vi "CreateSMGR_01_file_old.vi"(7 "file path to write":path, 8 "error in":errorcluster, 10 "Waveform Graph":waveform(i16)[](graph), 11 "meas_point":i32=4) -> (0 "error out":errorcluster, 1 "microseconds str":string, 2 "date str":string, 3 "file path out":path, 4 "max_values":string[](array[string]))   [LabVIEW 2010]
panel:
  out "dt":dbl format="%#_6f"
  out "max_value str":string
  # "Записываем данные в смешанном виде (текстовый/бинарный)\n-------------------------------------------------------------------------------\nСправка по формату лежит здесь\nhttp://smgr-devel.alwaysdata.net/doku.php?id=start\n\nЕсли включен дебаг, то в файл записываются две синусоиды\nа время ставится текущее"
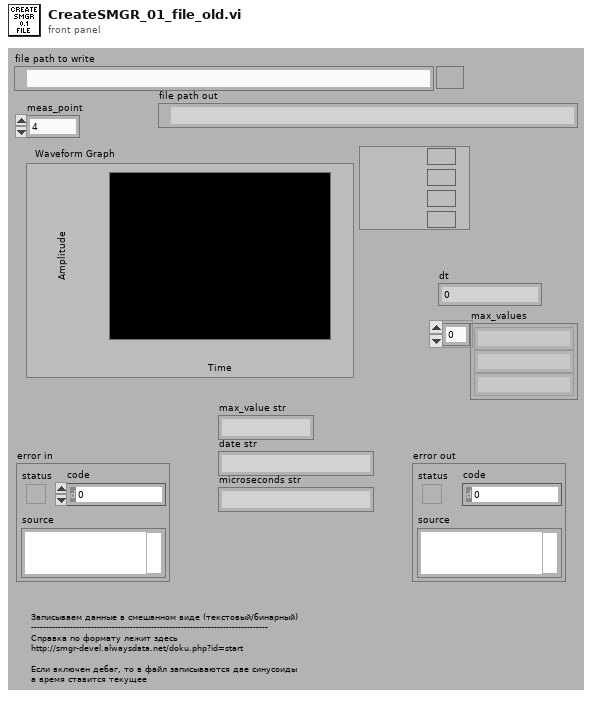
[diagram p1: front panel]
types:
  T1 = enum16{"sync", "phase_a", "phase_b", "phase_c", "ground"}
  T2 = enum16{"big-endian, network order", "native, host order", "little-endian"}
  T3 = enum16{"open", "replace", "create", "open or create", "replace or create", "replace or create with confirmation"}
  T4 = typedef "LVDateTimeRec.ctl" = cluster{"fractional second":dbl, "second":i32, "minute":i32, "hour":i32, "day of month":i32, "month":i32, "year":i32, "day of week":i32, "day of year":i32, "DST":i32}
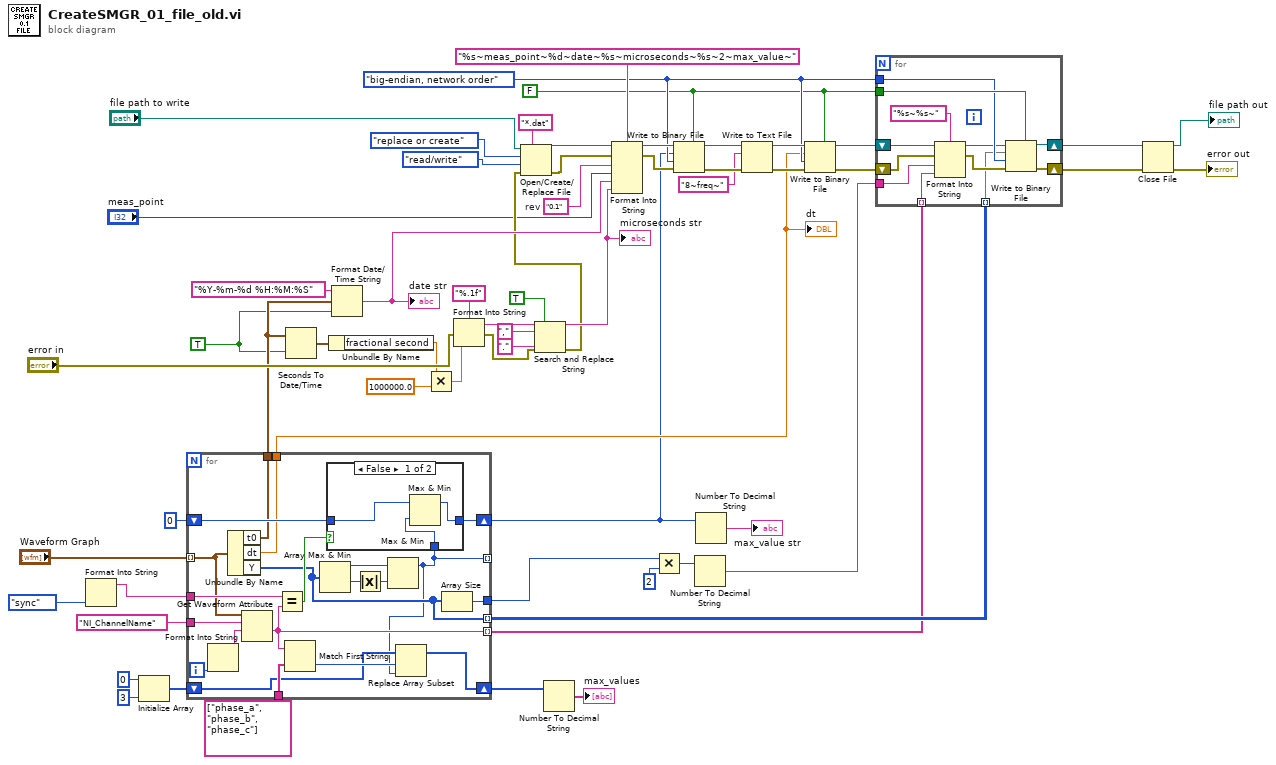
[diagram p0: block diagram]
diagram:
  w9 = TRUE ("to UTC (F)")
  w50 = "0.1"  # rev
  w39 = FALSE ("prepend array or string size? (T)")
  w40 = T2."big-endian, network order" ("byte order (0:big-endian, network order)")
  n1 = Format Into String(T1."sync") -> (resulting string=w16:string)  [unwired: 3 in, 1 out]
  n2 = Initialize Array(i16 0 ("element"), 3 ("dimension size")) -> (w4:i16[])
  n3 = for {
    tunnel: "Waveform Graph" -> [w78] mode=indexing
    tunnel: [w68] -> w41 mode=indexing
    tunnel: [w66] -> w8 mode=indexing
    shift-right: [w79] -> w3
    shift-left: i16 0 -> [w82]
    tunnel: w16 -> [w81]
    tunnel: "NI_ChannelName" -> [w77]
    tunnel: [w74] -> w15
    tunnel: [w73] -> w14
    tunnel: [w72] -> w13
    tunnel: [w62] -> _ mode=indexing
    tunnel: string[] ["phase_a", "phase_b", "phase_c"] -> [w67]
    shift-right: [w63] -> w2
    shift-left: w4 -> [w64]
    i -> [w76]
    n4 = Format Into String(w76) -> (resulting string=w75:string)  [unwired: 3 in, 1 out]
    n5 = Unbundle By Name(w78) -> ("t0"=w73:timestamp, "dt"=w74:dbl, "Y"=w68:i16[])
    n6 = Get Waveform Attribute(5:w75, 6:w77, 7:w78) -> (1:w66:string)  [unwired: 1 in, 3 out]
    n7 = Equal?(x=w81, y=w66) -> (x = y?=w80:bool)
    n8 = Match First String(2:w67, 3:w66) -> (0:w65:i32)  [unwired: 1 out]
    n9 = Array Max & Min(array=w68) -> (max value=w70:i16, min value=w69:i16)  [unwired: 2 out]
    n10 = Absolute Value(x=w69) -> (abs(x)=w71:i16)
    n11 = Max & Min(x=w70, y=w71) -> (max(x,y)=w62:i16)  [unwired: 1 out]
    n12 = case shown="False" w80 {
      tunnel: w82 -> [w84 w86]
      tunnel: [w85 w86] -> w79
      tunnel: w62 -> [w83 _]
      frame False {
        n13 = Max & Min(x=w84, y=w83) -> (max(x,y)=w85:i16)  [unwired: 1 out]
      }
      frame True {
      }
    }
    n14 = Replace Array Subset(array=w64, new element=w62, index=w65) -> (w63:i16[])
    n15 = Array Size(array=w68) -> (size(s)=w72:i32)
  }
  "dt" <- w15
  n16 = Seconds To Date/Time(time stamp (now)=w14, to UTC (F)=w9) -> (date time rec=w52:T4)
  n17 = Unbundle By Name(w52) -> ("fractional second"=w24:dbl)
  n18 = Format Date/Time String(time format string (%c)="%Y-%m-%d %H:%M:%S", seconds (now)=w14, UTC format=w9) -> (date/time string=w49:string)
  "date str" <- w49
  n19 = Multiply(x=w24, y=1000000.0) -> (x*y=w22:dbl)
  n20 = Format Into String(format string="%.1f", error in="error in", w22) -> (resulting string=w33:string, error out=w31:errorcluster)  [unwired: 1 in]
  n21 = Search and Replace String(replace all?=TRUE ("replace all? (F)"), input string=w33, search string=",", replace string="." ("replace string (\"\")"), error in=w31) -> (result string=w27:string, error out=w26:errorcluster)  [unwired: 3 in, 2 out]
  "microseconds str" <- w27
  n22 = Open/Create/Replace File(file path (use dialog)="file path to write", error in=w26, prompt="*.dat", operation (0:open)=T3."replace or create", access (0:read/write)=enum16{"read/write", "read-only", "write-only"}."read/write") -> (refnum out=w57:refnum<file>, error out=w56:errorcluster)  [unwired: 1 in, 1 out]
  n23 = Number To Decimal String(number=w2) -> (decimal integer string=→"max_values":string[])  [unwired: 1 in]
  n24 = Format Into String(format string="%s~meas_point~%d~date~%s~microseconds~%s~2~max_value~", initial string=w57, error in=w56, w50, "meas_point", w49, w27) -> (resulting string=w55:refnum<file>, error out=w54:errorcluster)
  n25 = Multiply(x=w13, y=2 ("index")) -> (x*y=w37:i32)
  n26 = Write to Binary File(file (use dialog)=w55, data=w3, error in=w54, 5:w39, 9:w40) -> (refnum out=w47:refnum<file>, error out=w48:errorcluster)  [unwired: 1 in, 1 out]
  n27 = Number To Decimal String(number=w37) -> (decimal integer string=w38:string)  [unwired: 1 in]
  n28 = Number To Decimal String(number=w3) -> (decimal integer string=→"max_value str":string)  [unwired: 1 in]
  n29 = Write to Text File(file (use dialog)=w47, text="8~freq~" ("prompt"), error in=w48) -> (refnum out=w45:refnum<file>, error out=w44:errorcluster)  [unwired: 1 in, 1 out]
  n30 = Write to Binary File(file (use dialog)=w45, data=w15, error in=w44, 5:w39, 9:w40) -> (refnum out=w43:refnum<file>, error out=w42:errorcluster)  [unwired: 1 in, 1 out]
  n31 = for {
    shift-right: [w91] -> w10
    shift-left: w43 -> [w98]
    shift-right: [w93] -> w11
    shift-left: w42 -> [w95]
    tunnel: w41 -> [w87] mode=indexing
    tunnel: w8 -> [w88] mode=indexing
    tunnel: w40 -> [w96]
    tunnel: w39 -> [w97]
    tunnel: w38 -> [w89]
    n32 = Format Into String(format string="%s~%s~" ("prompt"), initial string=w98, error in=w95, w89, w88) -> (resulting string=w92:refnum<file>, error out=w94:errorcluster)
    n33 = Write to Binary File(file (use dialog)=w92, data=w87, error in=w94, 5:w97, 9:w96) -> (refnum out=w91:refnum<file>, error out=w93:errorcluster)  [unwired: 1 in, 1 out]
  }
  n34 = Close File(refnum=w10, error in=w11) -> (path=→"file path out":path, error out=→"error out":errorcluster)
